vi "Receive.vi"(8 "error in (no error)":errorcluster, 9 "timeout in ms (-1)":i32=-1, 11 "DataSocketMessenger in":refnum<class "DataSocketMessenger.lvclass">) -> (0 "error out":errorcluster, 1 "timed out?":bool, 2 "Message":refnum<class "MSG.lvclass">, 3 "DataSocketMessenger out":refnum<class "DataSocketMessenger.lvclass">)   [LabVIEW 2011, in "Messenging.lvlib" / "DataSocketMessenger.lvclass"]
uses:
  DataSocketMessenger.lvclass
  TextVarientMessage/MSG.lvclass
  DataSocketMessenger.lvclass/DataSocketMessenger.ctl
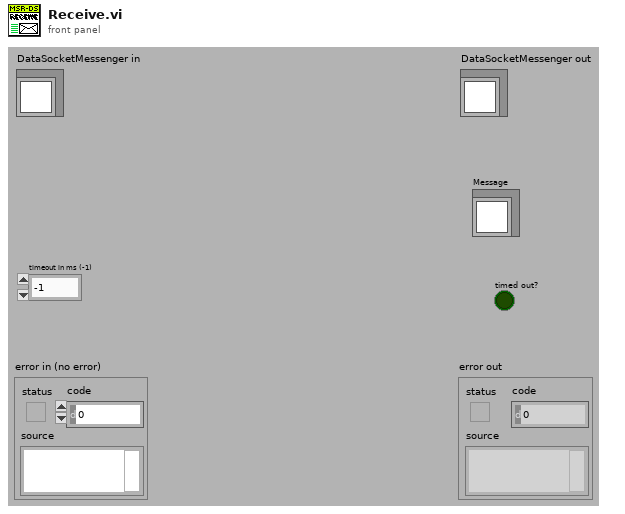
[diagram p1: front panel]
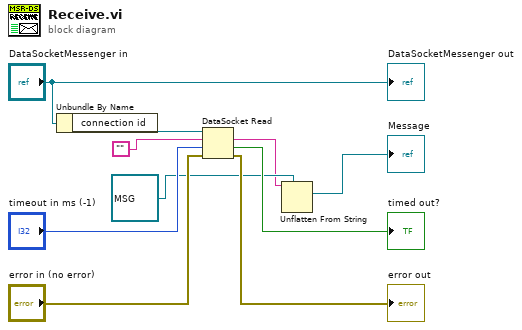
[diagram p0: block diagram]
diagram:
  n1 = Unbundle By Name("DataSocketMessenger in") -> ("connection id"=w10:refnum<k13>)
  n2 = DataSocket Read(8:"error in (no error)", 9:"timeout in ms (-1)", 10:"", 11:w10) -> (0:→"error out":errorcluster, 1:→"timed out?":bool, 2:w2:string)  [unwired: 5 out]
  n3 = Unflatten From String(type=refnum<class "MSG.lvclass"> refnum ("Message"), binary string=w2) -> (value=→"Message":refnum<class "MSG.lvclass">)  [unwired: 1 in, 4 out]
  "DataSocketMessenger out" <- "DataSocketMessenger in"
